vi "cube rotate.vi"(6 "cube rotation direction":T1, 8 "error in (no error)":errorcluster, 11 "cube in":T2) -> (0 "error out":errorcluster, 3 "cube out":T2)   [LabVIEW 2011]
uses:
  Typedef/cube.ctl
  Typedef/face.ctl
  Typedef/cube rotate direction.ctl
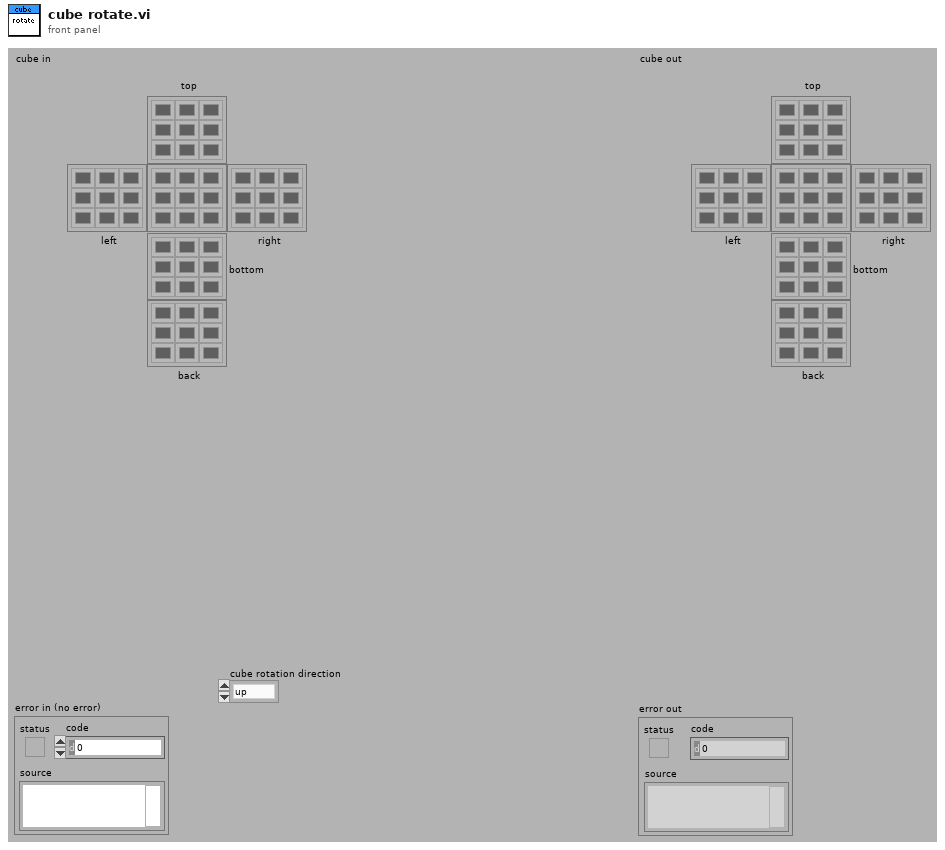
[diagram p1: front panel]
types:
  T1 = typedef "cube rotate direction.ctl" = enum16{"up", "down", "left", "right"}
  T2 = typedef "cube.ctl" = cluster{"top":T3, "left":T3, "right":T3, "bottom":T3, "back":T3, "front":T3}
  T3 = typedef "face.ctl" = u32[][]
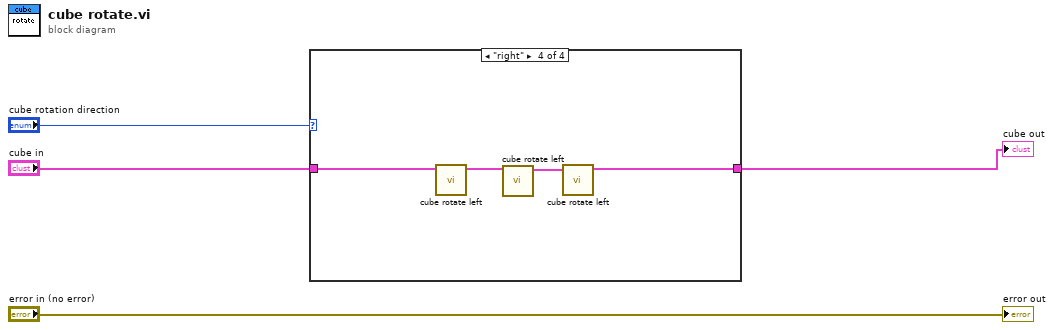
[diagram p0: block diagram]
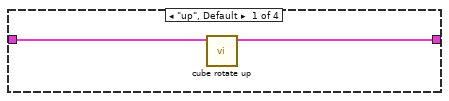
[diagram p2: hidden frame]
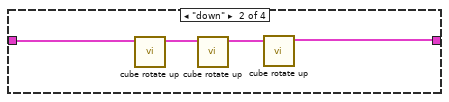
[diagram p3: hidden frame]
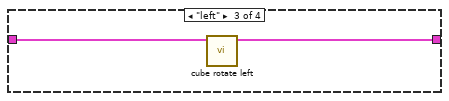
[diagram p4: hidden frame]
diagram:
  n1 = case shown="\"right\"" "cube rotation direction" {
    tunnel: [w6 w7 w12 w13] -> w4
    tunnel: "cube in" -> [w5 w10 w11 w16]
    frame "up", Default {
      n2 = call "cube rotate up.vi"("cube in"=w5) -> ("cube out"=w6:T2)  [unwired: 9 in, 1 out]
    }
    frame "down" {
      n3 = call "cube rotate up.vi"("cube in"=w10) -> ("cube out"=w9:T2)  [unwired: 9 in, 1 out]
      n4 = call "cube rotate up.vi"("cube in"=w9) -> ("cube out"=w8:T2)  [unwired: 9 in, 1 out]
      n5 = call "cube rotate up.vi"("cube in"=w8) -> ("cube out"=w7:T2)  [unwired: 9 in, 1 out]
    }
    frame "left" {
      n6 = call "cube rotate left.vi"("cube in"=w11) -> ("cube out"=w12:T2)  [unwired: 9 in, 1 out]
    }
    frame "right" {
      n7 = call "cube rotate left.vi"("cube in"=w16) -> ("cube out"=w15:T2)  [unwired: 9 in, 1 out]
      n8 = call "cube rotate left.vi"("cube in"=w15) -> ("cube out"=w14:T2)  [unwired: 9 in, 1 out]
      n9 = call "cube rotate left.vi"("cube in"=w14) -> ("cube out"=w13:T2)  [unwired: 9 in, 1 out]
    }
  }
  "cube out" <- w4
  "error out" <- "error in (no error)"
